vi "UPDATE MAPS.vi"(8 "Anticipate Graduation Year Map In":map{string, i32}(c390), 9 "Status Map In":map{string, i32}(c390), 10 "Department Map In":map{string, i32}(c390), 11 "REFERENCES":T1) -> (0 "Anticipate Graduation Year Map Out":map{string, i32}(c390), 1 "Status Map Out":map{string, i32}(c390), 2 "Department Map Out":map{string, i32}(c390))   [LabVIEW 2019]
uses:
  Controls/References Cluster.ctl
  <vilib>/userDefined/High Color/IMAQdx.ctl
  Controls/Custom Calendar/Custom Calendar.xctl
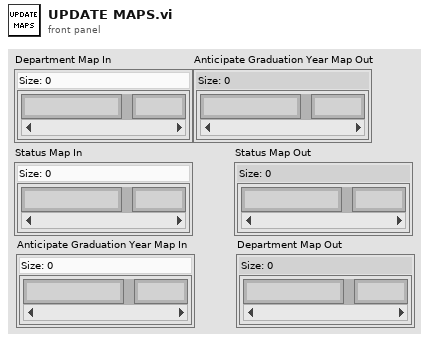
[diagram p1: front panel]
types:
  T1 = typedef "References Cluster.ctl" = cluster{"MAIN PAGES":refnum<vi>, "ADD/EDIT ITEM REFERENCES":cluster{"Identifier":refnum<vi>, "BYU ICN #":refnum<vi>, "Item Description":refnum<vi>, "Comments":refnum<vi>, "Checked Out Date":refnum<vi>, "Due Date":refnum<vi>, "Check Out Location":refnum<vi>, "Reminder Count":refnum<vi>, "Most Recent Reminder Date":refnum<vi>, "BYU ID #":refnum<vi>, "Building/Room":refnum<vi>, "Location in Room":refnum<vi>, "Manual":refnum<vi>, "Manufacturer":refnum<vi>, "Model #":refnum<vi>, "Serial #":refnum<vi>, "Date Acquired":refnum<vi>, "ADD/EDIT ITEM LABEL":refnum<vi>, "ARCHIVE ITEM":refnum<vi>, "Archive Item Inputs":refnum<vi>, "Reminder Notes":refnum<vi>}, "ADD/EDIT USER REFERENCES":cluster{"BYU ID # (##-###-####)":refnum<vi>, "First Name":refnum<vi>, "Last Name":refnum<vi>, "Phone Number (###-###-####)":refnum<vi>, "Email":refnum<vi>, "Department":refnum<vi>, "Graduation Status":refnum<vi>, "Anticipated Graduation Year":refnum<vi>, "Credit Score":refnum<vi>, "Date Added":refnum<vi>, "Graduation Clearance Date":refnum<vi>, "Picture File Name":refnum<vi>, "ADD/EDIT USER LABEL":refnum<vi>, "Department Map":refnum<vi>, "Status Map":refnum<vi>, "Anticipated Graduation Year Map":refnum<vi>, "User Agreement":refnum<vi>, "User Comments":refnum<vi>, "Camera":refnum<vi>}, "RETURN ITEM REFERENCES":cluster{"Item or Person:":refnum<vi>, "Search Return Results":refnum<vi>, "What are you searching for?":refnum<vi>}, "SEARCH DATABASE REFERENCES":cluster{"What to Search For:":refnum<vi>, "Where to Search":refnum<vi>, "Column to Search In":refnum<vi>, "Column to Sort By":refnum<vi>, "Search Database Results":refnum<vi>, "Inventory Column Selector":refnum<vi>, "User Column Selector":refnum<vi>, "Inventory Archive Column Selector":refnum<vi>, "User Archive Column Selector":refnum<vi>, "Sales Tracking Column Selector":refnum<vi>, "Checked In Archive Column Selector":refnum<vi>, "Restore User":refnum<vi>, "Date Range":refnum<vi>, "Dates Less Than":refnum<vi>, "Dates Greater Than":refnum<vi>, "Search Print Receipt":refnum<vi>}, "USER ITEMS REFERENCES":cluster{"USER'S INFORMATION":refnum<vi>, "User's Checked Out Items":refnum<vi>, "User Info Comments":refnum<vi>, "SEE USER INFO COMMENTS":refnum<vi>}, "EDIT ITEMS REFERENCES":cluster{"New Check Out Location":refnum<vi>, "Items to Edit":refnum<vi>, "Edit Items Due Date":refnum<vi>, "New Reminder Notes":refnum<vi>, "New Item Description":refnum<vi>}, "CHECK OUT ITEMS REFERENCES":cluster{"Enter Item:":refnum<vi>, "Check Out Items Due Date":refnum<vi>, "Check Out Location":refnum<vi>, "Items to be Checked Out":refnum<vi>, "Possible Items":refnum<vi>}, "TRANSFER ITEMS REFERENCES":cluster{"Search Parameter":refnum<vi>, "What to Match":refnum<vi>, "Matching Individuals":refnum<vi>, "Items to be Transferred":refnum<vi>}, "SETTINGS REFERENCES":cluster{"PSC Database Settings":refnum<vi>, "PSC Sales Item Spreadsheet":refnum<vi>}, "PSC SALES REFERENCES":cluster{"BYU ID CARD #":refnum<vi>, "Sale Description":refnum<vi>, "Scan or Enter Item Name":refnum<vi>, "Items to be Sold":refnum<vi>, "Grand Total":refnum<vi>, "Item List":refnum<vi>}}
  T2 = typedef "LVStringsAndValuesArrayTypeDef_U16.ctl" = cluster{"String":string, "Value":u16}[]
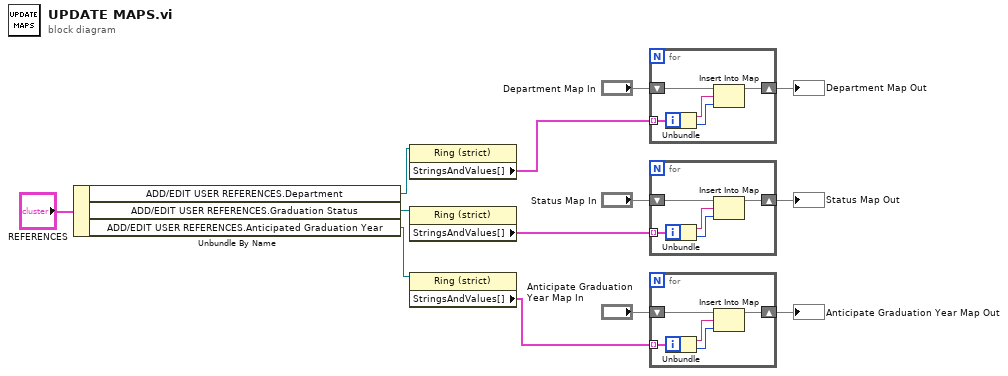
[diagram p0: block diagram]
diagram:
  n1 = Unbundle By Name("REFERENCES") -> ("ADD/EDIT USER REFERENCES.Department"=w12:refnum<vi>, "ADD/EDIT USER REFERENCES.Graduation Status"=w11:refnum<vi>, "ADD/EDIT USER REFERENCES.Anticipated Graduation Year"=w10:refnum<vi>)
  n2 = property class="Ring (strict)"(reference=w12) -> ("StringsAndValues[]"=w9:T2)  [unwired: 1 in, 2 out]
  n3 = property class="Ring (strict)"(reference=w11) -> ("StringsAndValues[]"=w7:T2)  [unwired: 1 in, 2 out]
  n4 = property class="Ring (strict)"(reference=w10) -> ("StringsAndValues[]"=w3:T2)  [unwired: 1 in, 2 out]
  n5 = for {
    tunnel: w9 -> [w18] mode=indexing
    shift-right: [w14] -> w6
    shift-left: "Department Map In" -> [w17]
    n6 = Unbundle(w18) -> ("String"=w16:string, "Value"=w15:u16)
    n7 = Insert Into Map(map in=w17, key=w16, value=w15) -> (map out=w14:map{string, i32})  [unwired: 2 out]
  }
  "Department Map Out" <- w6
  n8 = for {
    tunnel: w7 -> [w23] mode=indexing
    shift-right: [w19] -> w4
    shift-left: "Status Map In" -> [w22]
    n9 = Unbundle(w23) -> ("String"=w21:string, "Value"=w20:u16)
    n10 = Insert Into Map(map in=w22, key=w21, value=w20) -> (map out=w19:map{string, i32})  [unwired: 2 out]
  }
  "Status Map Out" <- w4
  n11 = for {
    tunnel: w3 -> [w28] mode=indexing
    shift-right: [w24] -> w1
    shift-left: "Anticipate Graduation Year Map In" -> [w27]
    n12 = Unbundle(w28) -> ("String"=w26:string, "Value"=w25:u16)
    n13 = Insert Into Map(map in=w27, key=w26, value=w25) -> (map out=w24:map{string, i32})  [unwired: 2 out]
  }
  "Anticipate Graduation Year Map Out" <- w1
